vi "String.Append 1D to String List.vi"(5 "1DDelimiter":string=";", 7 "GroupDelimiter":string="| ", 10 "New 1D Data":string[](array[string]), 11 "Existing Str":string) -> (3 "New Str":string)   [LabVIEW 2019]
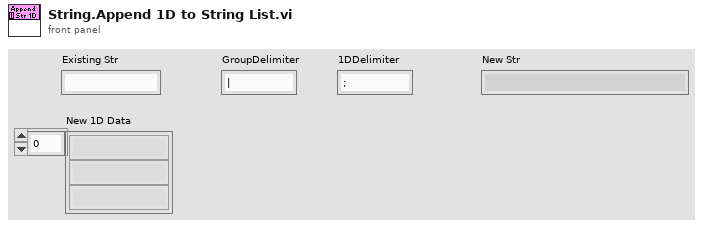
[diagram p1: front panel]
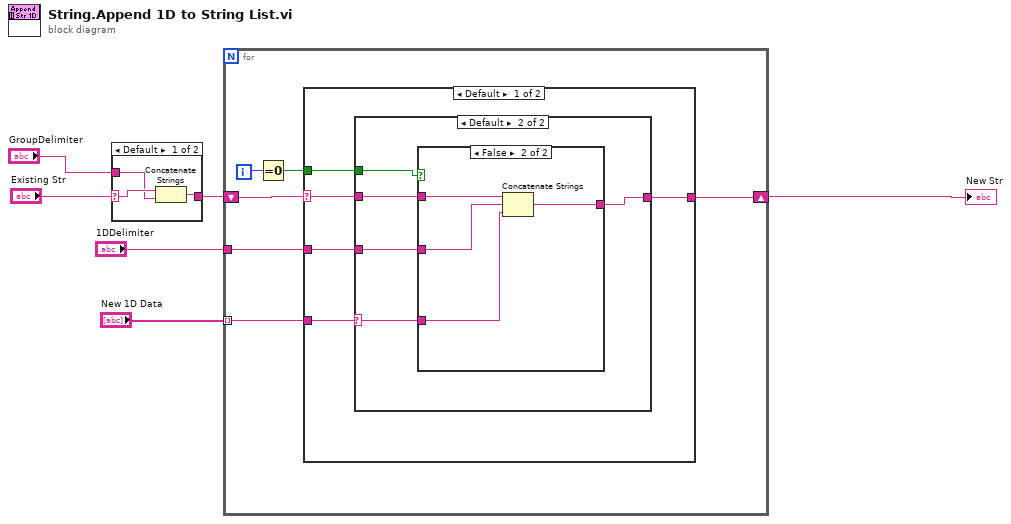
[diagram p0: block diagram]
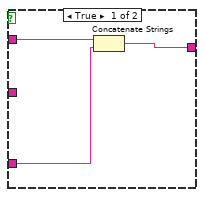
[diagram p4: hidden frame]
diagram:
  n1 = case shown="Default" "Existing Str" {
    selector: "Existing Str" -> [w9 w10]
    tunnel: "GroupDelimiter" -> [w8 _]
    tunnel: [w7 w10] -> w1
    frame Default {
      n2 = Concatenate Strings(w9, w8) -> (w7:string)
    }
    frame "\u0000" {
    }
  }
  n3 = for {
    tunnel: "New 1D Data" -> [w14] mode=indexing
    tunnel: "1DDelimiter" -> [w13]
    shift-right: [w15] -> w4
    shift-left: w1 -> [w16]
    i -> [w12]
    n4 = Equal To 0?(x=w12) -> (x = 0?=w11:bool)
    n5 = case shown="Default" w16 {
      selector: w16 -> [w21 _]
      tunnel: [w19 w35] -> w15
      tunnel: w14 -> [w20 w35]
      tunnel: w13 -> [w18 _]
      tunnel: w11 -> [w17 _]
      frame Default {
        n6 = case shown="Default" w20 {
          selector: w20 -> [_ w26]
          tunnel: w21 -> [w22 w27]
          tunnel: [w22 w25] -> w19
          tunnel: w18 -> [_ w24]
          tunnel: w17 -> [_ w23]
          frame "" {
          }
          frame Default {
            n7 = case shown="False" w23 {
              tunnel: w27 -> [w30 w31]
              tunnel: w26 -> [w29 w34]
              tunnel: [w28 w33] -> w25
              tunnel: w24 -> [_ w32]
              frame True {
                n8 = Concatenate Strings(w30, w29) -> (w28:string)
              }
              frame False {
                n9 = Concatenate Strings(w31, w32, w34) -> (w33:string)
              }
            }
          }
        }
      }
      frame "" {
      }
    }
  }
  "New Str" <- w4
